vi "WriteOutTagFiles.vi"(5 "SimpleDataset":bool, 8 "error IN":errorcluster, 9 "file path (use dialog)":path, 10 "TagList":string[](array[string]), 11 "SimplePosTable":string[][](array[string])) -> (0 "ErrorArray":errorcluster[](array[cluster]))   [LabVIEW 2011]
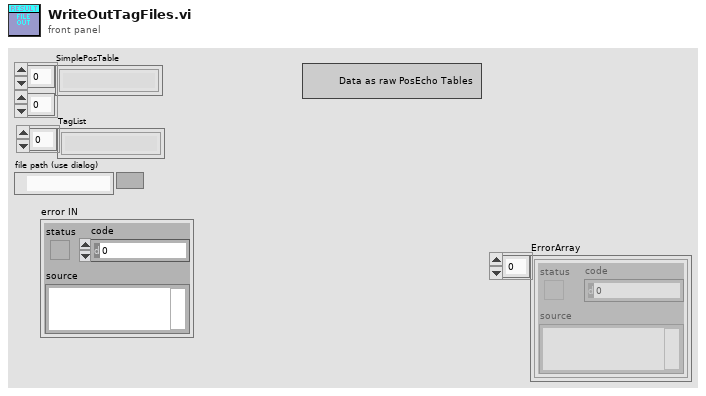
[diagram p1: front panel]
types:
  T1 = enum16{"open", "replace", "create", "open or create", "replace or create", "replace or create with confirmation"}
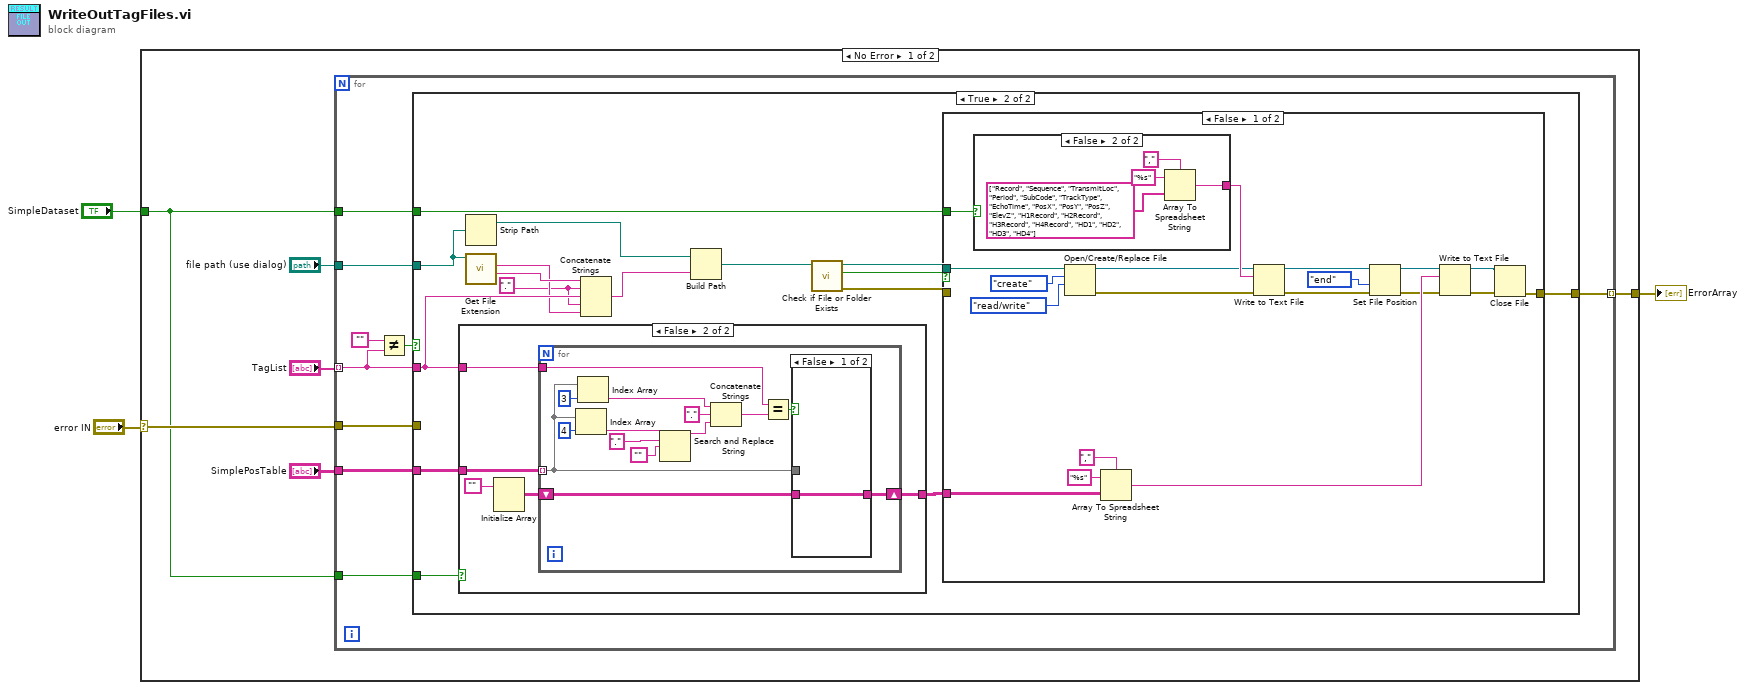
[diagram p0: block diagram]
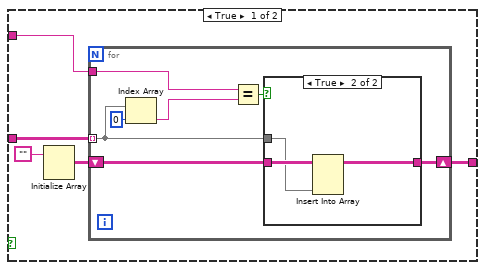
[diagram p3: hidden frame]
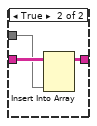
[diagram p5: hidden frame]
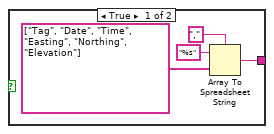
[diagram p6: hidden frame]
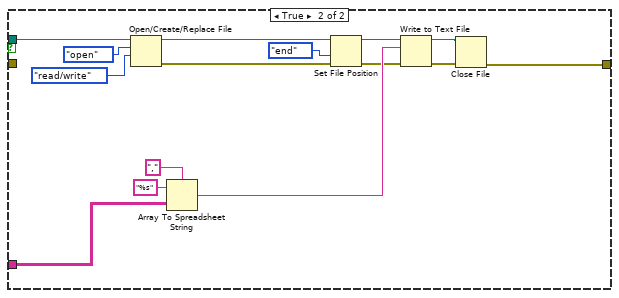
[diagram p7: hidden frame]
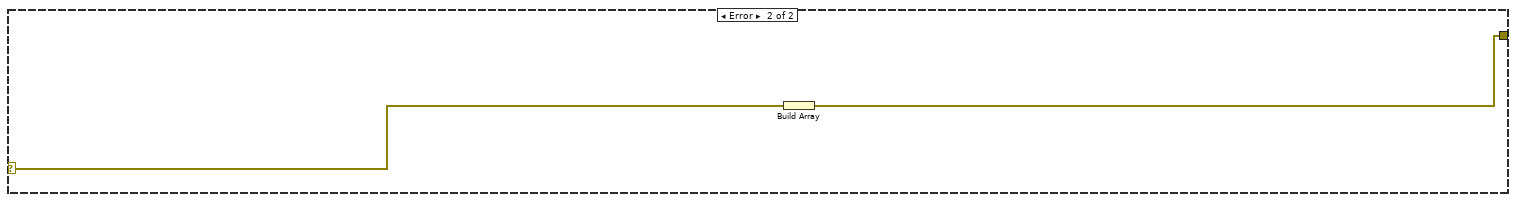
[diagram p8: hidden frame]
diagram:
  n1 = case shown="No Error" "error IN" {
    selector: "error IN" -> [w5 w118]
    tunnel: [w6 w117] -> w3
    tunnel: "SimpleDataset" -> [w4 _]
    frame No Error {
      n2 = for {
        tunnel: "TagList" -> [w14] mode=indexing
        tunnel: "SimplePosTable" -> [w18]
        tunnel: "file path (use dialog)" -> [w17]
        tunnel: [w16] -> w6 mode=indexing
        tunnel: w5 -> [w12]
        tunnel: w4 -> [w11]
        tunnel: w4 -> [w10]
        n3 = Not Equal?(x="", y=w14) -> (x != y?=w15:bool)
        n4 = case shown="True" w15 {
          tunnel: w18 -> [_ w35]
          tunnel: w17 -> [_ w34]
          tunnel: w14 -> [_ w31]
          tunnel: [w19 w24] -> w16
          tunnel: w12 -> [w19 _]
          tunnel: w11 -> [_ w21]
          tunnel: w10 -> [_ w20]
          frame False {
          }
          frame True {
            w22 = "." ("string")
            n5 = case shown="False" w20 {
              tunnel: w35 -> [w40 w56]
              tunnel: w31 -> [w37 w53]
              tunnel: [w36 w52] -> w25
              frame True {
                n6 = Initialize Array("") -> (w38:string[][])  [unwired: 2 in]
                n7 = for {
                  tunnel: w40 -> [w41] mode=indexing
                  tunnel: w37 -> [w45]
                  shift-right: [w42] -> w36
                  shift-left: w38 -> [w43]
                  n8 = Index Array(array=w41, index=0) -> (element=w46:string)
                  n9 = Equal?(x=w45, y=w46) -> (x = y?=w44:bool)
                  n10 = case shown="True" w44 {
                    tunnel: w43 -> [w48 w50]
                    tunnel: [w48 w51] -> w42
                    tunnel: w41 -> [_ w49]
                    frame False {
                    }
                    frame True {
                      n11 = Insert Into Array(array=w50, new element=w49) -> (w51:string[][])  [unwired: 2 in]
                    }
                  }
                }
              }
              frame False {
                n12 = Initialize Array("") -> (w54:string[][])  [unwired: 2 in]
                n13 = for {
                  tunnel: w56 -> [w65] mode=indexing
                  tunnel: w53 -> [w69]
                  shift-right: [w66] -> w52
                  shift-left: w54 -> [w67]
                  n14 = Index Array(array=w65, index=4) -> (element=w60:string)
                  n15 = Index Array(array=w65, index=3) -> (element=w57:string)
                  n16 = Search and Replace String(input string=w60, search string=".", replace string="") -> (result string=w58:string)  [unwired: 5 in, 3 out]
                  n17 = Concatenate Strings(w57, "." ("string"), w58) -> (w64:string)
                  n18 = Equal?(x=w69, y=w64) -> (x = y?=w68:bool)
                  n19 = case shown="False" w68 {
                    tunnel: w67 -> [w71 w73]
                    tunnel: [w71 w74] -> w66
                    tunnel: w65 -> [_ w72]
                    frame False {
                    }
                    frame True {
                      n20 = Insert Into Array(array=w73, new element=w72) -> (w74:string[][])  [unwired: 2 in]
                    }
                  }
                }
              }
            }
            n21 = Strip Path(path=w34) -> (stripped path=w33:path)  [unwired: 1 out]
            n22 = call <vilib>:"Get File Extension.vi"("file"=w34) -> ("filename without extension"=w32:string, "lowercase file extension"=w23:string)  [unwired: 7 in, 2 out]
            n23 = Concatenate Strings(w32, w22, w31, w22, w23) -> (w30:string)
            n24 = Build Path(base path=w33, name or relative path=w30) -> (appended path=w29:path)
            n25 = call <vilib>:"Check if File or Folder Exists.vi"("path"=w29) -> ("error out"=w27:errorcluster, "file or folder exists?"=w26:bool, "dup path"=w28:path)  [unwired: 8 in]
            n26 = case shown="False" w26 {
              tunnel: w28 -> [w88 w114]
              tunnel: w27 -> [_ _]
              tunnel: w25 -> [w85 w111]
              tunnel: [w76 w104] -> w24
              tunnel: w21 -> [w75 _]
              frame False {
                n27 = case shown="False" w75 {
                  tunnel: [w95 w99] -> w93
                  frame True {
                    n28 = Array To Spreadsheet String(delimiter (Tab)=",", array=string[] ["Tag", "Date", "Time", "Easting", "Northing", "Elevation"] ("Array"), 3:"%s" ("format string")) -> (spreadsheet string=w95:string)
                  }
                  frame False {
                    n29 = Array To Spreadsheet String(delimiter (Tab)=",", array=string[] ["Record", "Sequence", "TransmitLoc", "Period", "SubCode", "TrackType", "EchoTime", "PosX", "PosY", "PosZ", "ElevZ", "H1Record", "H2Record", "H3Record", "H4Record", "HD1", "HD2", "HD3", "HD4"] ("Array"), 3:"%s" ("format string")) -> (spreadsheet string=w99:string)
                  }
                }
                n30 = Open/Create/Replace File(file path (use dialog)=w88, operation (0:open)=T1."create", access (0:read/write)=enum16{"read/write", "read-only", "write-only"}."read/write") -> (refnum out=w91:refnum<file>, error out=w92:errorcluster)  [unwired: 3 in, 1 out]
                n31 = Array To Spreadsheet String(delimiter (Tab)=",", array=w85, 3:"%s" ("format string")) -> (spreadsheet string=w81:string)
                n32 = Write to Text File(file (use dialog)=w91, text=w93, error in=w92) -> (refnum out=w83:refnum<file>, error out=w82:errorcluster)  [unwired: 1 in, 1 out]
                n33 = Set File Position(refnum=w83, from (0:start)=enum16{"start", "end", "current"}."end", error in=w82) -> (refnum out=w80:refnum<file>, error out=w79:errorcluster)  [unwired: 1 in]
                n34 = Write to Text File(file (use dialog)=w80, text=w81, error in=w79) -> (refnum out=w78:refnum<file>, error out=w77:errorcluster)  [unwired: 1 in, 1 out]
                n35 = Close File(refnum=w78, error in=w77) -> (error out=w76:errorcluster)  [unwired: 1 out]
              }
              frame True {
                n36 = Open/Create/Replace File(file path (use dialog)=w114, operation (0:open)=T1."open", access (0:read/write)=enum16{"read/write", "read-only", "write-only"}."read/write") -> (refnum out=w103:refnum<file>, error out=w102:errorcluster)  [unwired: 3 in, 1 out]
                n37 = Array To Spreadsheet String(delimiter (Tab)=",", array=w111, 3:"%s" ("format string")) -> (spreadsheet string=w109:string)
                n38 = Set File Position(refnum=w103, from (0:start)=enum16{"start", "end", "current"}."end", error in=w102) -> (refnum out=w108:refnum<file>, error out=w107:errorcluster)  [unwired: 1 in]
                n39 = Write to Text File(file (use dialog)=w108, text=w109, error in=w107) -> (refnum out=w106:refnum<file>, error out=w105:errorcluster)  [unwired: 1 in, 1 out]
                n40 = Close File(refnum=w106, error in=w105) -> (error out=w104:errorcluster)  [unwired: 1 out]
              }
            }
          }
        }
      }
    }
    frame Error {
      n41 = Build Array(w118) -> (w117:errorcluster[])
    }
  }
  "ErrorArray" <- w3
